vi "Defragment TDMS.vi"() -> ()   [LabVIEW 2018]
uses:
  <vilib>/Utility/sysdir.llb/System Directory Type.ctl
panel:
  out "Default data 2":path
  out "Tmp":path
  out "Default data":path
  in  "File Path Control":path
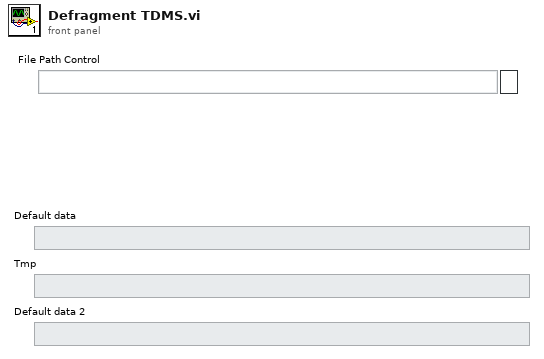
[diagram p1: front panel]
types:
  T1 = typedef "System Directory Type.ctl" = i32
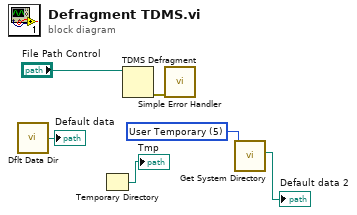
[diagram p0: block diagram]
diagram:
  w2 = T1 5 items=["User Home"=0, "User Desktop"=1, "User Documents"=2, "User Application Data"=3, "User Preferences"=4, "User Temporary"=5, "Public Documents"=6, "Public Application Data"=7, "Public Preferences"=8, "Public Cache"=13, "System Core Libraries"=9, "System Installed Libraries"=10, "Application Files"=11, "Boot Volume Root"=12] ("system directory type")
  n1 = call <vilib>:"Dflt Data Dir.vi"() -> ("App:Default Data Directory"=→"Default data":path)
  n2 = Temporary Directory() -> (→"Tmp":path)
  n3 = TDMS Defragment(7:"File Path Control") -> (0:w6:errorcluster)  [unwired: 1 in]
  n4 = call <vilib>:"Simple Error Handler.vi"("error in (no error)"=w6) -> ()  [unwired: 4 in, 5 out]
  n5 = call <vilib>:"Get System Directory.vi"("system directory type"=w2) -> ("system directory"=→"Default data 2":path)  [unwired: 10 in]
